vi "Write Error Log.vi"(0 "Session Handle in":T1, 5 "Process Name":string, 7 "Data":string, 11 "error in (no error)":errorcluster) -> (4 "Session Handle out":T1, 15 "error out":errorcluster)   [LabVIEW 2015, in "Circular Error Log.lvclass"]
uses:
  Circular Error Log.lvclass
  Typedefs/Session Handle.ctl
  Circular Error Log.lvclass/Circular Error Log.ctl
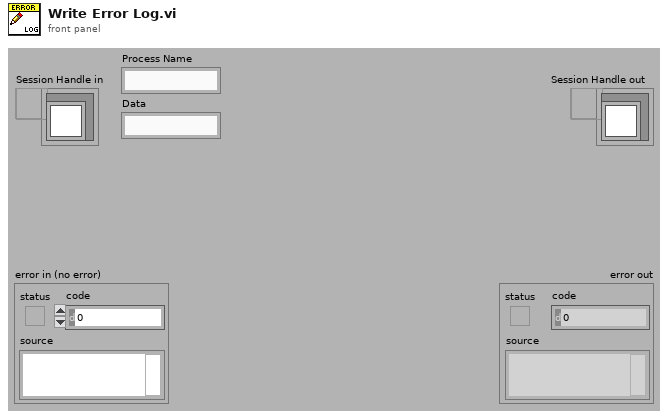
[diagram p1: front panel]
types:
  T1 = typedef "Circular Error Log.lvclass/Session Handle.ctl" = refnum<data-value>
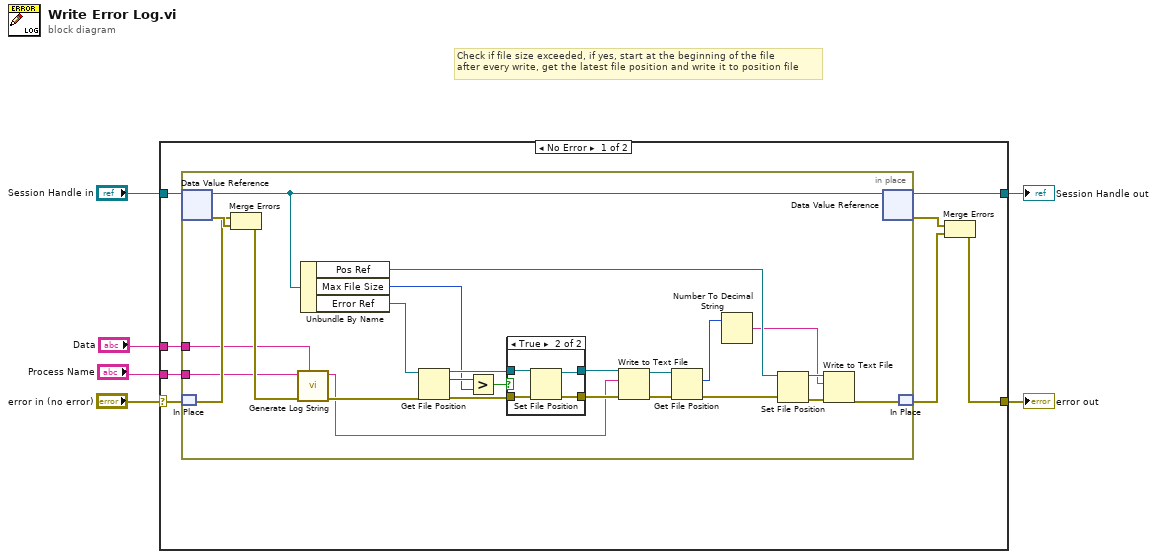
[diagram p0: block diagram]
diagram:
  # "Check if file size exceeded, if yes, start at the beginning of the file\nafter every write, get the latest file position and write it to position file"
  n1 = case shown="No Error" "error in (no error)" {
    selector: "error in (no error)" -> [w9 w46]
    tunnel: "Session Handle in" -> [w14 w47]
    tunnel: [w13 w47] -> w5
    tunnel: [w10 w46] -> w4
    tunnel: "Process Name" -> [w8 _]
    tunnel: "Data" -> [w7 _]
    frame No Error {
      n2 = in-place {
        in-place-border: w8 -> [w36]
        in-place-border: w7 -> [w35]
        n3 = in-place-dvr #1(w14) -> (w24:refnum<class "Circular Error Log.lvclass">, w39:errorcluster)
        n4 = in-place-match #2(w9) -> (w38:errorcluster)
        n5 = Merge Errors(w38, w39) -> (w37:errorcluster)
        n6 = call "Generate Log String.vi"("Log"=w35, "error in (no error)"=w37, "Process Name"=w36) -> ("error out"=w28:errorcluster, "Log String"=w25:string)  [unwired: 7 in]
        n7 = Unbundle By Name(w24) -> ("Pos Ref"=w21:refnum<file>, "Max File Size"=w26:i64, "Error Ref"=w27:refnum<file>)
        n8 = Get File Position(4:w28, 7:w27) -> (0:w31:errorcluster, 2:w34:i64, 3:w32:refnum<file>)
        n9 = Greater?(x=w34, y=w26) -> (0:w33:bool)
        n10 = case shown="True" w33 {
          tunnel: w31 -> [w41 w45]
          tunnel: w32 -> [w40 w44]
          tunnel: [w41 w43] -> w30
          tunnel: [w40 w42] -> w29
          frame False {
          }
          frame True {
            n11 = Set File Position(refnum=w44, error in=w45) -> (refnum out=w42:refnum<file>, error out=w43:errorcluster)  [unwired: 2 in]
          }
        }
        n12 = Write to Text File(file (use dialog)=w29, text=w25, error in=w30) -> (refnum out=w23:refnum<file>, error out=w22:errorcluster)  [unwired: 1 in, 1 out]
        n13 = Get File Position(4:w22, 7:w23) -> (0:w15:errorcluster, 2:w17:i64)  [unwired: 1 out]
        n14 = Number To Decimal String(number=w17) -> (decimal integer string=w16:string)  [unwired: 1 in]
        n15 = Set File Position(refnum=w21, error in=w15) -> (refnum out=w20:refnum<file>, error out=w19:errorcluster)  [unwired: 2 in]
        n16 = Write to Text File(file (use dialog)=w20, text=w16, error in=w19) -> (error out=w18:errorcluster)  [unwired: 1 in, 2 out]
        n17 = in-place-dvr #1(w24) -> (w13:T1, w11:errorcluster)
        n18 = in-place-match #2(w18) -> (w12:errorcluster)
      }
      n19 = Merge Errors(w11, w12) -> (w10:errorcluster)
    }
    frame Error {
    }
  }
  "Session Handle out" <- w5
  "error out" <- w4
